vi "Pump 4 RT FIFO.vi"(0 "Data IN":u16[](array[numeric]), 1 "Mode (Write)":T1=enum."Write", 7 "Buffer Size":i32=10, 9 "# of elements":i32=1, 11 "Error IN":errorcluster) -> (4 "Data OUT":u16[][](array[numeric]), 15 "Error OUT":errorcluster)   [LabVIEW 2019]
uses:
  Real-Time/Controls/RT FIFO Mode.ctl
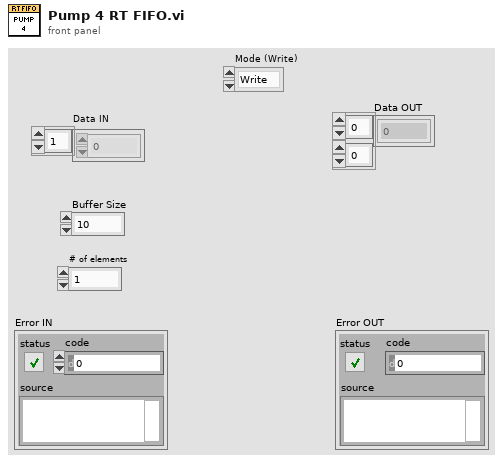
[diagram p1: front panel]
types:
  T1 = typedef "RT FIFO Mode.ctl" = enum16{"Create", "Write", "Read", "Delete"}
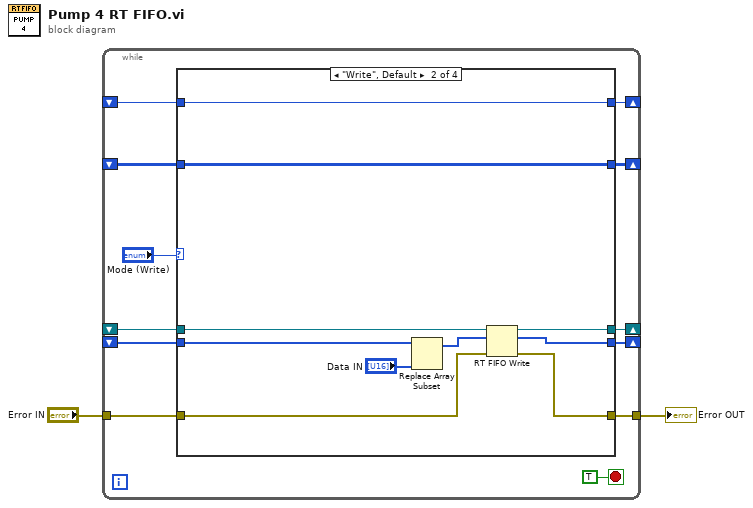
[diagram p0: block diagram]
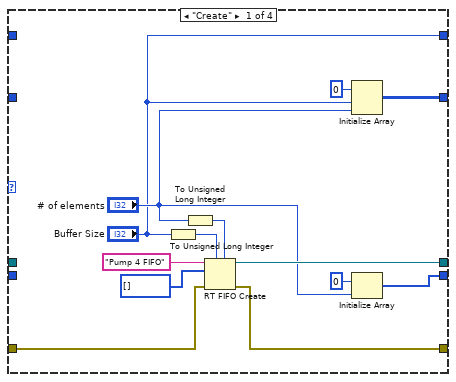
[diagram p2: hidden frame]
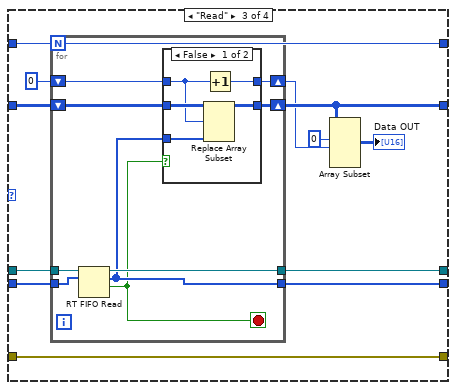
[diagram p3: hidden frame]
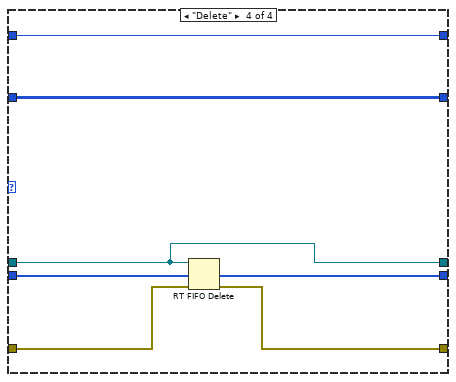
[diagram p5: hidden frame]
diagram:
  n1 = while {
    shift-right: [w12] -> _
    shift-left: _ -> [w11]
    tunnel: "Error IN" -> [w10]
    tunnel: [w9] -> w1
    shift-right: [w8] -> _
    shift-left: _ -> [w7]
    shift-right: [w6] -> _
    shift-left: _ -> [w5]
    shift-right: [w4] -> _
    shift-left: _ -> [w3]
    stop <- TRUE stop-if-true
    n2 = case shown="\"Write\", Default" "Mode (Write)" {
      tunnel: [w26 w35 w46 w70] -> w12
      tunnel: w11 -> [_ w36 w47 w70]
      tunnel: w10 -> [w22 w32 w48 w68]
      tunnel: [w21 w31 w48 w67] -> w9
      tunnel: [w23 w33 w44 w69] -> w8
      tunnel: w7 -> [_ w34 w45 w69]
      tunnel: [w16 w30 w41 w66] -> w6
      tunnel: w5 -> [_ w30 w42 w66]
      tunnel: ["Buffer Size" w29 w37 w65] -> w4
      tunnel: w3 -> [_ w29 w37 w65]
      frame "Create" {
        n3 = To Unsigned Long Integer(number="Buffer Size") -> (unsigned 32bit integer=w17:u32)
        n4 = To Unsigned Long Integer(number="# of elements") -> (unsigned 32bit integer=w20:u32)
        n5 = RT FIFO Create(0:"Pump 4 FIFO" ("name (unnamed)"), 1:u16[] [], 3:w22, 4:w17, 6:w20) -> (8:w26:refnum<k33>, 11:w21:errorcluster)  [unwired: 3 in, 1 out]
        n6 = Initialize Array(u16 0, "Buffer Size", "# of elements") -> (w16:u16[][])
        n7 = Initialize Array(u16 0, "# of elements") -> (w23:u16[])
      }
      frame "Write", Default {
        n8 = Replace Array Subset(array=w34, new element="Data IN") -> (w33:u16[])  [unwired: 1 in]
        n9 = RT FIFO Write(0:w36, 1:w33, 3:w32) -> (8:w35:refnum<k33>, 11:w31:errorcluster)  [unwired: 2 in, 2 out]
      }
      frame "Read" {
        n10 = for {
          N: w37 -> [_]
          tunnel: w47 -> [w57]
          tunnel: [w56] -> w46
          tunnel: w45 -> [w55]
          tunnel: [w50] -> w44
          shift-right: [w53] -> w39
          shift-left: 0 -> [w54]
          shift-right: [w51] -> w41
          shift-left: w42 -> [w52]
          stop <- w49 stop-if-true
          n11 = RT FIFO Read(0:w57, 1:w55) -> (8:w56:refnum<k33>, 9:w50:u16[], 10:w49:bool)  [unwired: 2 in, 2 out]
          n12 = case shown="False" w49 {
            tunnel: w54 -> [w59 w64]
            tunnel: [w62 w64] -> w53
            tunnel: w52 -> [w61 w63]
            tunnel: [w60 w63] -> w51
            tunnel: w50 -> [w58 _]
            frame False {
              n13 = Replace Array Subset(array=w61, new element=w58, index (row)=w59) -> (w60:u16[][])  [unwired: 1 in]
              n14 = Increment(x=w59) -> (x+1=w62:i32)
            }
            frame True {
            }
          }
        }
        n15 = Array Subset(array=w41, index (row)=0 ("index"), length (row)=w39) -> (→"Data OUT":u16[][])  [unwired: 2 in]
      }
      frame "Delete" {
        n16 = RT FIFO Delete(0:w70, 3:w68) -> (11:w67:errorcluster)  [unwired: 1 in]
      }
    }
  }
  "Error OUT" <- w1
